vi "Read Pulse Parameters.vi"(8 "error in (no error)":errorcluster, 11 "RFSoC Driver in":refnum<class "RFSoC Driver.lvclass">) -> (0 "error out":errorcluster, 2 "Pulse Parameters":T1={"clock rate"=1200000000.0, "Frequency"=217000000.0, "NWaves"=75, "standard deviation"=0.1, "Amplitude"=32767.0, "Mode"=enum."Sine"} {"Frequency" format="%#_6pHz"; "clock rate" format="%#_6pHz"}, 3 "RFSoC Driver out":refnum<class "RFSoC Driver.lvclass">)   [LabVIEW 2020, in "RFSoC Driver.lvclass"]
uses:
  RFSoC Driver.lvclass
  Pulse Parameters.ctl
  RFSoC Driver.lvclass/RFSoC Driver.ctl
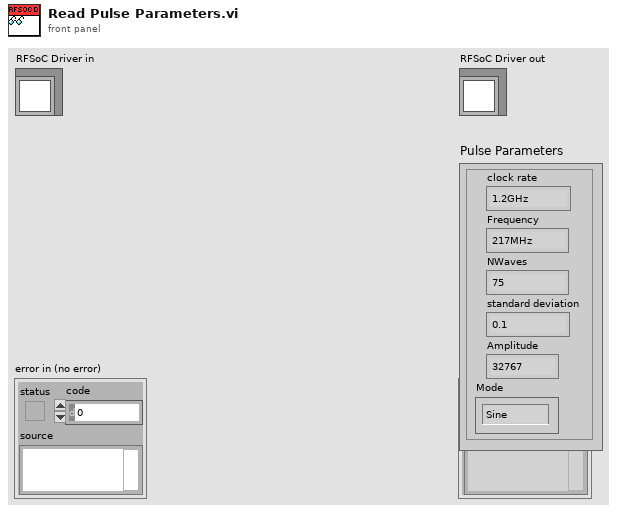
[diagram p1: front panel]
types:
  T1 = typedef "Pulse Parameters.ctl" = cluster{"clock rate":dbl, "Frequency":dbl, "NWaves":i32, "standard deviation":dbl, "Amplitude":dbl, "Mode":enum16{"Sine", "Pulse"}}
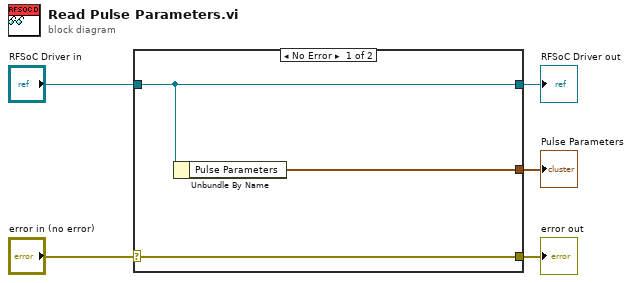
[diagram p0: block diagram]
diagram:
  n1 = case shown="No Error" "error in (no error)" {
    selector: "error in (no error)" -> [w8 w9]
    tunnel: [w8 w9] -> w4
    tunnel: [w7 w10] -> w2
    tunnel: "RFSoC Driver in" -> [w7 w10]
    tunnel: [w6 _] -> w1
    frame No Error {
      n2 = Unbundle By Name(w7) -> ("Pulse Parameters"=w6:T1)
    }
    frame Error {
    }
  }
  "error out" <- w4
  "RFSoC Driver out" <- w2
  "Pulse Parameters" <- w1
